vi "niLvFpga_WriteFifo_cRIO-9043.vi"(0 "session in":u32, 1 "ScalarType":u32=4294967295, 2 "BitWidth":u32=4294967295, 5 "Channel":u32, 7 "Data":u32[](array[numeric]), 11 "error in":errorcluster, 12 "Timeout(ms)":i32=-1) -> (4 "session out":u32, 10 "Sample Backlog":u32, 15 "error out":errorcluster)   [LabVIEW 2017]
doc: "Performance related peculiarities:\n\n1. Disable the Call Library Function's \"Generate Wrappers\" feature. This feature is displayed when you add the following labview.ini token, and right click on the Call Library Function node:\nextFuncGenNoWrapperEnabled=True\n\n2. For the Call Library function, enable \"Constant\" for parameters >> session.\n\n3. Remove the error case structure around the Call Library Functions. Chaining the errors between multiple Call Library Functions will suffice."
uses:
  <vilib>/rvi/errors/niLvFpgaWhatHappensToTopLevelVI.ctl
  <vilib>/rvi/interface/common/niFpgaNodeNameForErrorReporting.ctl
  <vilib>/rvi/interface/common/niFpgaWaitOnOcc.vi
  NiFpgaLv.dll
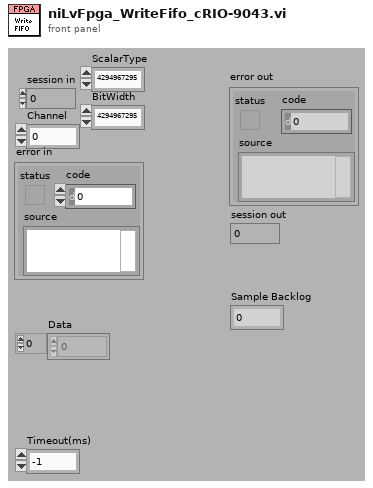
[diagram p1: front panel]
types:
  T1 = typedef "niFpgaNodeNameForErrorReporting.ctl" = enum16{"Open FPGA VI Reference", "Read/Write Control", "Invoke Method: Abort", "Invoke Method: Acknowledge IRQ", "Invoke Method: Download", "Invoke Method: FIFO.Configure", "Invoke Method: FIFO.Read", "Invoke Method: FIFO.Start", "Invoke Method: FIFO.Stop", "Invoke Method: FIFO.Write", "Invoke Method: Reset", "Invoke Method: Run", "Invoke Method: Wait on IRQ", "Close FPGA VI Reference", "Invoke Method: FIFO.Acquire Read Region", "Invoke Method: FIFO.Acquire Write Region"}
  T2 = typedef "niLvFpgaWhatHappensToTopLevelVI.ctl" = enum16{"top level VI scripted behind XNode", "top level VI inlined behind XNode"}
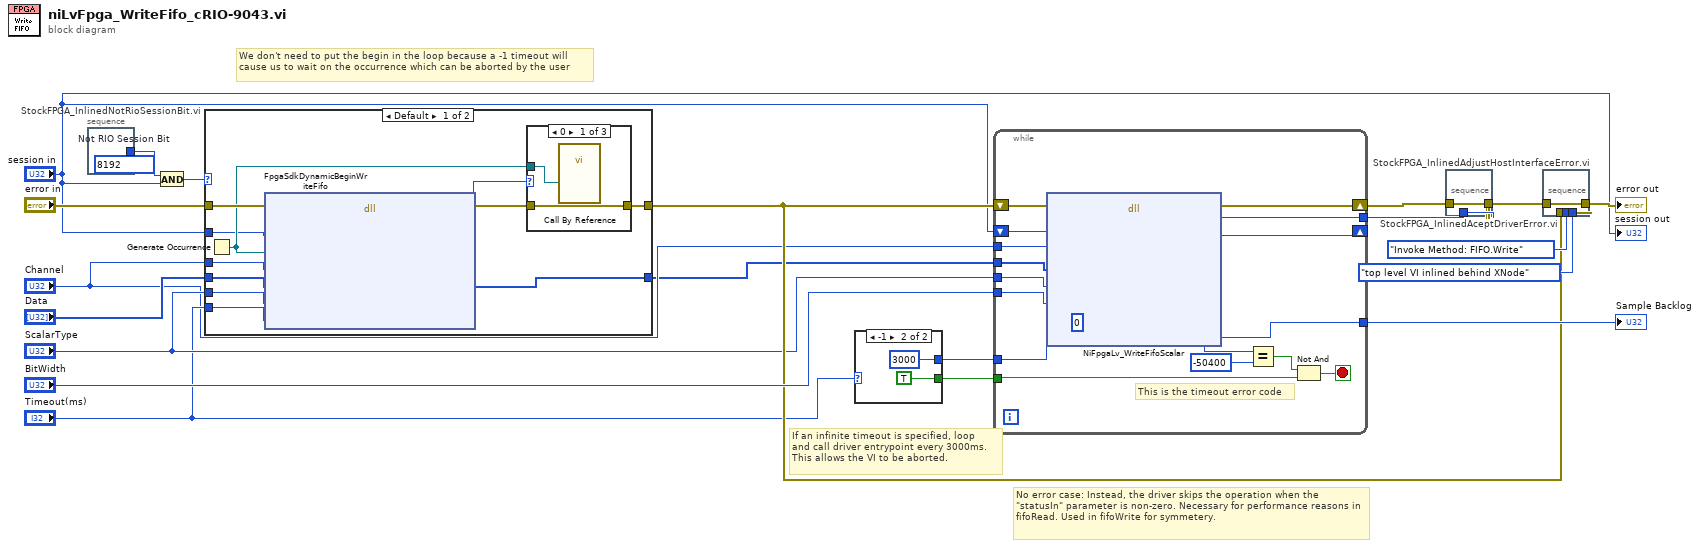
[diagram p0: block diagram]
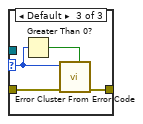
[diagram p5: hidden frame]
diagram:
  # "We don't need to put the begin in the loop because a -1 timeout will cause us to wait on the occurrence which can be aborted by the user"
  # "No error case: Instead, the driver skips the operation when the \"statusIn\" parameter is non-zero. Necessary for performance reasons in fifoRead. Used in fifoWrite for symmetery."
  # "If an infinite timeout is specified, loop\nand call driver entrypoint every 3000ms.\nThis allows the VI to be aborted."
  n1 = stacked-sequence "StockFPGA_InlinedNotRioSessionBit.vi" {
    tunnel: [w21] -> w9
    frame #0 {
      w21 = u32 8192  # Not RIO Session Bit
    }
  }
  n2 = And(x=w9, y="session in") -> (x .and. y?=w10:u32)
  n3 = case shown="Default" w10 {
    tunnel: "error in" -> [w31 w41]
    tunnel: [w32 w41] -> w7
    tunnel: "session in" -> [w28 _]
    tunnel: "Channel" -> [w27 _]
    tunnel: "Data" -> [w26 w40]
    tunnel: "ScalarType" -> [w25 _]
    tunnel: "Timeout(ms)" -> [w24 _]
    tunnel: [w22 w40] -> w1
    frame Default {
      n4 = Generate Occurrence() -> (w29:refnum<k4>)
      n5 = dll-call lib="LabVIEW" fn="FpgaSdkDynamicBeginWriteFifo"(error in=w31, "session"=w28, "occurrence"=w29, "channel"=w27, "Data"=w26, "scalarType"=w25, "timeout"=w24) -> (error out=w30:errorcluster, "status"=w23:i32, "Data"=w22:u32[])  [unwired: 7 in, 1 out]
      n6 = case shown="0" w23 {
        selector: w23 -> [_ _ w37]
        tunnel: [w34 w35 w39] -> w32
        tunnel: w29 -> [w33 _ _]
        tunnel: w30 -> [w34 w35 w36]
        frame 0 {
          n7 = call-by-ref "?"("occurrence"=w33) -> ()  [unwired: 16 in, 3 out]
        }
        frame -61167 {
          # "emulation case intentionally ignoring error"
        }
        frame Default {
          n8 = Greater Than 0?(x=w37) -> (x > 0?=w38:bool)
          n9 = call <vilib>:"Error Cluster From Error Code.vi"("is warning? (False)"=w38, "error in (no error)"=w36, "error code (0)"=w37) -> ("error out"=w39:errorcluster)  [unwired: 6 in]
        }
      }
    }
    frame 0 {
    }
  }
  n10 = case shown="-1" "Timeout(ms)" {
    selector: "Timeout(ms)" -> [w42 _]
    tunnel: [w42 3000] -> w19
    tunnel: [_ TRUE] -> w20
    frame Default {
    }
    frame -1 {
    }
  }
  n11 = while {
    tunnel: [w53] -> w18
    tunnel: w20 -> [w57]
    tunnel: w19 -> [w54]
    tunnel: "Channel" -> [w55]
    tunnel: [w51] -> w17
    shift-right: [w50] -> _
    shift-left: "session in" -> [w56]
    tunnel: w1 -> [w49]
    shift-right: [w47] -> w13
    shift-left: w7 -> [w48]
    tunnel: "ScalarType" -> [w46]
    tunnel: "BitWidth" -> [w45]
    stop <- w58 stop-if-true
    # "This is the timeout error code"
    n12 = dll-call lib="NiFpgaLv.*" fn="NiFpgaLv_WriteFifoScalar" label="niLvFpgaWriteFifo"(error in=w48, "sessionID"=w56, "channel"=w55, "dataIn"=w49, "scalarType"=w46, "bitWidth"=w45, "timeout"=w54, "remaining"=u32 0 ("elementsRemaining")) -> (error out=w47:errorcluster, "status"=w53:i32, "sessionID"=w50:u32, "remaining"=w51:u32)  [unwired: 7 in, 1 out]
    n13 = Equal?(x=w53, y=-50400) -> (x = y?=w59:bool)
    n14 = Not And(1:w57, 2:w59) -> (0:w58:bool)
  }
  "Sample Backlog" <- w17
  n15 = stacked-sequence "StockFPGA_InlinedAceptDriverError.vi" {
    tunnel: w13 -> [w61]
    tunnel: w18 -> [w63]
    tunnel: [w62] -> w15
    frame #0 {
      n16 = case shown="Default" w63 {
        selector: w63 -> [_ w65]
        tunnel: [w64 w67] -> w62
        tunnel: w61 -> [w64 w68]
        frame 0 {
        }
        frame Default {
          n17 = Greater Than 0?(x=w65) -> (x > 0?=w66:bool)
          n18 = call <vilib>:"Error Cluster From Error Code.vi"("is warning? (False)"=w66, "error in (no error)"=w68, "error code (0)"=w65) -> ("error out"=w67:errorcluster)  [unwired: 6 in]
        }
      }
    }
  }
  n19 = stacked-sequence "StockFPGA_InlinedAdjustHostInterfaceError.vi" {
    tunnel: w15 -> [w74]
    tunnel: w7 -> [w71]
    tunnel: niFpgaNodeNameForErrorReporting."Invoke Method: FIFO.Write" ("node name for error reporting") -> [w69]
    tunnel: niLvFpgaWhatHappensToTopLevelVI."top level VI inlined behind XNode" ("what happens to top level VI") -> [w70]
    tunnel: [w72] -> w14
    frame #0 {
      n20 = Unbundle By Name(w74) -> ("code"=w73:i32)
      n21 = case shown="Default" w73 {
        tunnel: [w75 w80] -> w72
        tunnel: w71 -> [w75 w79]
        tunnel: w70 -> [_ w78]
        tunnel: w69 -> [_ w77]
        tunnel: w74 -> [_ w76]
        frame 0 {
        }
        frame Default {
          n22 = call <vilib>:"niLvFpgaAdjustHostInterfaceError.vi"("error in"=w76, "prior error in"=w79, "node name for error reporting"=w77, "what happens to top level VI"=w78) -> ("error out"=w80:errorcluster)  [unwired: 11 in]
        }
      }
    }
  }
  "error out" <- w14
  "session out" <- "session in"
